vi "Panel - Manual Control.vi"() -> ()   [LabVIEW 2020]
doc: "Panel to hold all manual controls"
uses:
  Library - Test Executive.llb/Test Executive - Globals.vi
panel:
  in  "Power Up":bool
  in  "Power Down":bool
  in  "Test":u16(ring) items=["1 Current Consumption", "2 Firmware Revision", "3 Indicators", "4 Gain", "5 Sensitivity"]
  in  "Run Single Test":bool
  in  "stop":bool
  in  "Check Test Equipment":bool
  in  "Power Up":bool
  in  "Power Down":bool
  in  "Reset All":bool
  out "errors":errorcluster
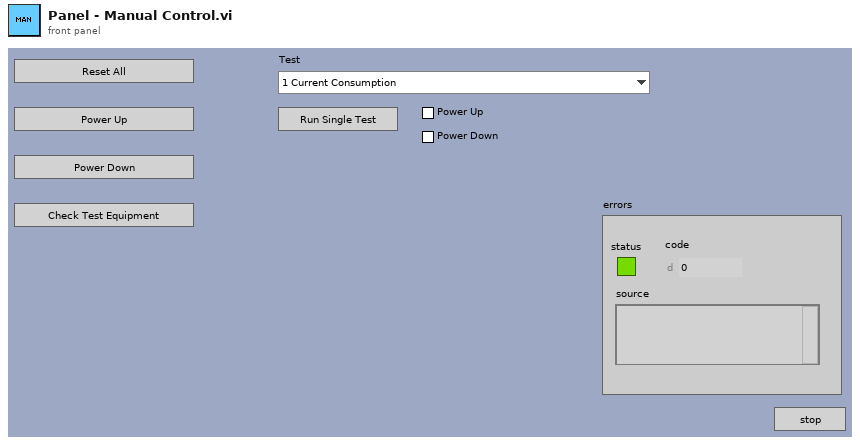
[diagram p1: front panel]
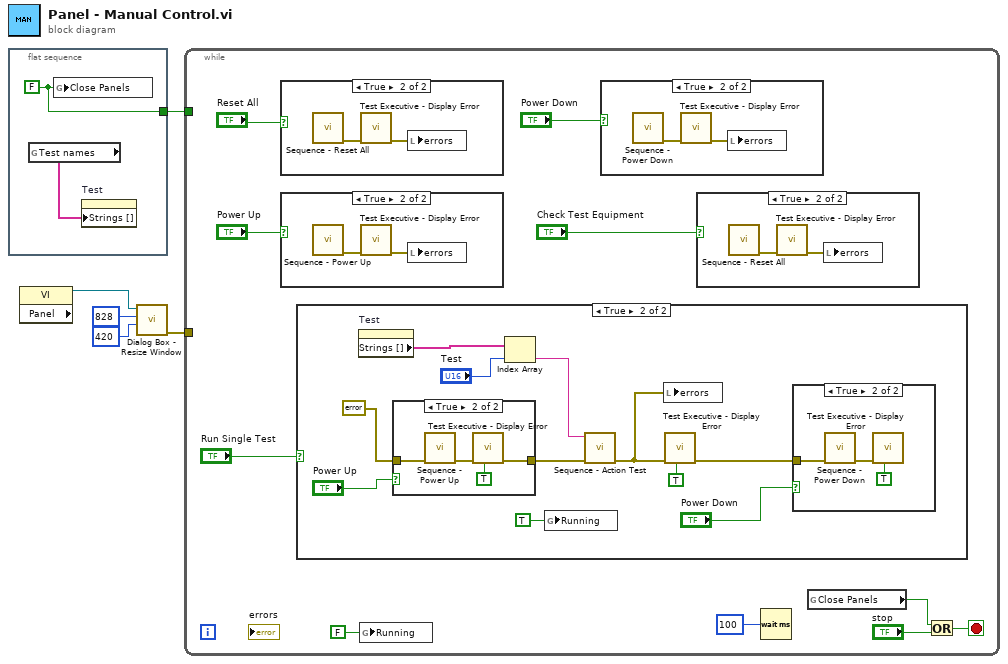
[diagram p0: block diagram]
diagram:
  n1 = flat-sequence {
    tunnel: [w7] -> w5
    frame #0 {
      w7 = FALSE ("Close Panels")
      n2 = global read "Test Executive - Globals.vi" "Test names"() -> (w6:string[])
      n3 = global write "Test Executive - Globals.vi" "Close Panels"(w7) -> ()
      n4 = property on="Test" class="Ring (strict)"("Strings []"=w6) -> ()  [unwired: 2 in, 2 out]
    }
  }
  n5 = property class="VI" props=["Panel"]() -> (reference out=w2:refnum<vi>)  [unwired: 2 in, 2 out]
  n6 = call "Dialog Box - Resize Window.vi"("Height"=i16 420, "Width"=i16 828, "reference"=w2) -> ("error out"=w1:errorcluster)  [unwired: 8 in]
  n7 = while {
    tunnel: w5 -> [_]
    tunnel: w1 -> [_]
    stop <- w11 stop-if-true
    n8 = case shown="True" "Reset All" {
      frame False {
      }
      frame True {
        n9 = call "Sequence - Reset All.vi"() -> ("error out"=w44:errorcluster)  [unwired: 11 in]
        n10 = call "Test Executive - Display Error.vi"("error in (no error)"=w44) -> ("error out"=w43:errorcluster)  [unwired: 10 in]
        n11 = local write "errors"(w43) -> ()
      }
    }
    n12 = case shown="True" "Power Up" {
      frame False {
      }
      frame True {
        n13 = call "Sequence - Power Up.vi"() -> ("error out"=w38:errorcluster)  [unwired: 11 in]
        n14 = call "Test Executive - Display Error.vi"("error in (no error)"=w38) -> ("error out"=w37:errorcluster)  [unwired: 10 in]
        n15 = local write "errors"(w37) -> ()
      }
    }
    n16 = case shown="True" "Run Single Test" {
      frame False {
      }
      frame True {
        n17 = property on="Test" class="Ring (strict)"() -> ("Strings []"=w23:string[])  [unwired: 2 in, 2 out]
        n18 = case shown="True" "Power Up" {
          tunnel: errorcluster {"status"=FALSE, "code"=0, "source"=""} ("error in (no error)") -> [w32 w36]
          tunnel: [w32 w35] -> w25
          frame False {
          }
          frame True {
            n19 = call "Sequence - Power Up.vi"("error in (no error)"=w36) -> ("error out"=w34:errorcluster)  [unwired: 10 in]
            n20 = call "Test Executive - Display Error.vi"("Clear Error"=TRUE, "error in (no error)"=w34) -> ("error out"=w35:errorcluster)  [unwired: 9 in]
          }
        }
        n21 = Index Array(array=w23, index="Test") -> (element=w22:string)
        n22 = global write "Test Executive - Globals.vi" "Running"(TRUE ("Running")) -> ()
        n23 = call "Sequence - Action Test.vi"("error in (no error)"=w25, "Test"=w22) -> ("error out"=w18:errorcluster)  [unwired: 9 in]
        n24 = local write "errors"(w18) -> ()
        n25 = call "Test Executive - Display Error.vi"("Clear Error"=TRUE, "error in (no error)"=w18) -> ("error out"=w19:errorcluster)  [unwired: 9 in]
        n26 = case shown="True" "Power Down" {
          tunnel: w19 -> [_ w31]
          frame False {
          }
          frame True {
            n27 = call "Sequence - Power Down.vi"("error in (no error)"=w31) -> ("error out"=w30:errorcluster)  [unwired: 10 in]
            n28 = call "Test Executive - Display Error.vi"("Clear Error"=TRUE, "error in (no error)"=w30) -> ()  [unwired: 9 in, 1 out]
          }
        }
      }
    }
    n29 = global write "Test Executive - Globals.vi" "Running"(FALSE ("Running")) -> ()
    n30 = case shown="True" "Power Down" {
      frame False {
      }
      frame True {
        n31 = call "Sequence - Power Down.vi"() -> ("error out"=w42:errorcluster)  [unwired: 11 in]
        n32 = call "Test Executive - Display Error.vi"("error in (no error)"=w42) -> ("error out"=w41:errorcluster)  [unwired: 10 in]
        n33 = local write "errors"(w41) -> ()
      }
    }
    n34 = case shown="True" "Check Test Equipment" {
      frame False {
      }
      frame True {
        n35 = call "Sequence - Reset All.vi"() -> ("error out"=w40:errorcluster)  [unwired: 11 in]
        n36 = call "Test Executive - Display Error.vi"("error in (no error)"=w40) -> ("error out"=w39:errorcluster)  [unwired: 10 in]
        n37 = local write "errors"(w39) -> ()
      }
    }
    n38 = Wait (ms)(milliseconds to wait=u32 100) -> ()  [unwired: 1 out]
    n39 = global read "Test Executive - Globals.vi" "Close Panels"() -> (w12:bool)
    n40 = Or(x=w12, y="stop") -> (x .or. y?=w11:bool)
  }
